vi "GenFromFile.vi"() -> ()   [LabVIEW 2017]
uses:
  <vilib>/sound2/lvsound2.llb/Sampling Mode.ctl
  <vilib>/sound2/lvsound2.llb/Sound File Info (path).vi
  <vilib>/sound2/lvsound2.llb/Sound File Read Open.vi
  <vilib>/sound2/lvsound2.llb/Sound File Read (DBL).vi
  <vilib>/sound2/lvsound2.llb/Sound Output Write (DBL).vi
panel:
  in  "number of samples/ch":i32=100000
  in  "stop":bool
  in  "path":path
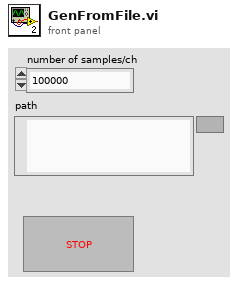
[diagram p1: front panel]
types:
  T1 = typedef "Sampling Mode.ctl" = i32
  T2 = typedef "Sound Data Format.ctl" = cluster{"sample rate (S/s)":dbl, "number of channels":i32, "bits per sample":i32}
  T3 = typedef "Sound Output Task ID.ctl" = u32
  T4 = typedef "Sound File Refnum.ctl" = refnum<file>
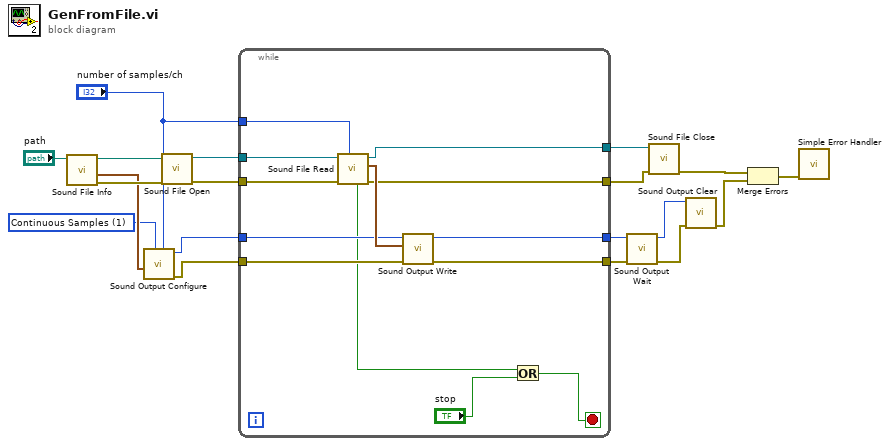
[diagram p0: block diagram]
diagram:
  w15 = T1 1 items=["Finite Samples", "Continuous Samples"] ("sample mode")
  n1 = call-poly <vilib>:"Sound File Info.vi"("path"="path") -> ("error out"=w17:errorcluster, "sound format"=w16:T2, "path out"=w18:path)  [unwired: 7 in, 1 out]
  n2 = call <vilib>:"Sound Output Configure.vi"("number of samples/ch"="number of samples/ch", "sample mode"=w15, "sound format"=w16) -> ("error out"=w11:errorcluster, "task ID"=w12:T3)  [unwired: 7 in]
  n3 = call-poly <vilib>:"Sound File Open.vi"("error in (no error)"=w17, "path"=w18) -> ("error out"=w13:errorcluster, "sound file refnum"=w14:T4)  [unwired: 8 in]
  n4 = while {
    tunnel: w14 -> [w32]
    tunnel: w13 -> [w31]
    tunnel: w12 -> [w29]
    tunnel: w11 -> [w28]
    tunnel: [w27] -> w3
    tunnel: [w26] -> w4
    tunnel: [w25] -> w10
    tunnel: [w24] -> w9
    tunnel: "number of samples/ch" -> [w20]
    stop <- w21 stop-if-true
    n5 = call-poly <vilib>:"Sound File Read.vi"("number of samples/ch (-1: all)"=w20, "error in (no error)"=w31, "sound file refnum"=w32) -> ("error out"=w24:errorcluster, "data"=w30:waveform(dbl)[], "sound file refnum out"=w25:T4, "end of file?"=w23:bool)  [unwired: 4 in, 1 out]
    n6 = call-poly <vilib>:"Sound Output Write.vi"("error in (no error)"=w28, "data"=w30, "task ID"=w29) -> ("error out"=w27:errorcluster, "task ID out"=w26:T3)  [unwired: 7 in]
    n7 = Or(x=w23, y="stop") -> (x .or. y?=w21:bool)
  }
  n8 = call <vilib>:"Sound Output Wait.vi"("error in (no error)"=w3, "task ID"=w4) -> ("error out"=w1:errorcluster, "task ID out"=w2:T3)  [unwired: 8 in]
  n9 = call <vilib>:"Sound File Close.vi"("error in (no error)"=w9, "sound file refnum"=w10) -> ("error out"=w8:errorcluster)  [unwired: 9 in]
  n10 = call <vilib>:"Sound Output Clear.vi"("error in (no error)"=w1, "task ID"=w2) -> ("error out"=w7:errorcluster)  [unwired: 9 in]
  n11 = Merge Errors(w8, w7) -> (w6:errorcluster)
  n12 = call <vilib>:"Simple Error Handler.vi"("error in (no error)"=w6) -> ()  [unwired: 4 in, 5 out]
